vi "Close Application.vi"(11 "VI in":refnum<vi>) -> ()   [LabVIEW 2020]
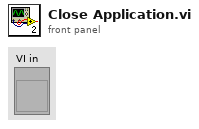
[diagram p1: front panel]
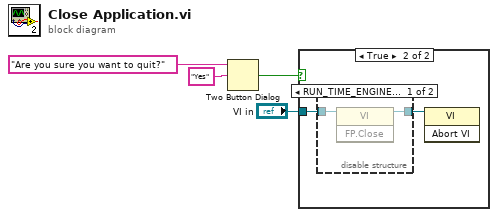
[diagram p0: block diagram]
diagram:
  n1 = Two Button Dialog(message="Are you sure you want to quit?", 2:"Yes" ("T button name (\"OK\")")) -> (T button?=w3:bool)  [unwired: 1 in]
  n2 = case shown="True" w3 {
    tunnel: "VI in" -> [_ w6]
    frame False {
    }
    frame True {
      n3 = disable-structure shown="RUN_TIME_ENGINE==True" {
        disable-tunnel: w6 -> [w8 w9]
        disable-tunnel: [w7 w9] -> w5
        frame condition #0 {
          n4 = invoke class="VI" method="FP.Close"(reference=w8) -> (reference out=w7:refnum<vi>)  [unwired: 2 in, 2 out]
        }
        frame condition #1 (active) {
        }
      }
      n5 = invoke class="VI" method="Abort VI"(reference=w5) -> ()  [unwired: 2 in, 3 out]
    }
  }
